vi "AxSyncLabVIEW.vi"() -> ()   [LabVIEW 2020]
panel:
  in  "Move position":i32
  in  "Refresh":bool
  in  "Tab Control":T1(tab)
  out "Analogue I/O":string
  out "Controller Type":string
  out "System Version":string
  out "Digital I/O":string
  out "Axis Parameters":string[][](table)
  in  "Axis":sgl
  out "HEX Representation of IO":string
  in  "WriteTable":bool
  in  "Entries":i32
  in  "Start":i32
  in  "Table Values":string[][](table)
  out "Table Size":dbl
  out "VR Values":string[][](table)
  in  "Start VR":ext
  in  "Entries VR":ext
  in  "Set VR":bool
  out "Directory Contents":string
  out "Status":string
  out "Axis Parameters 2":string[][](table)
  out "Watch Dog":bool
  in  "Run":bool
  out "CommPort":fxp<+,3,3>
  out "IsOpenLED":bool
  in  "Set Parameters":bool
  in  "Connection":string(combo)
  in  "Open/ Close":bool
  in  "stop":bool
  out "Error Out":errorcluster
  in  "Error In (no error)":errorcluster
  in  "Connection":refnum<k7>(container)
  # "WDOG OFF is illuminated\nas per coordinator"
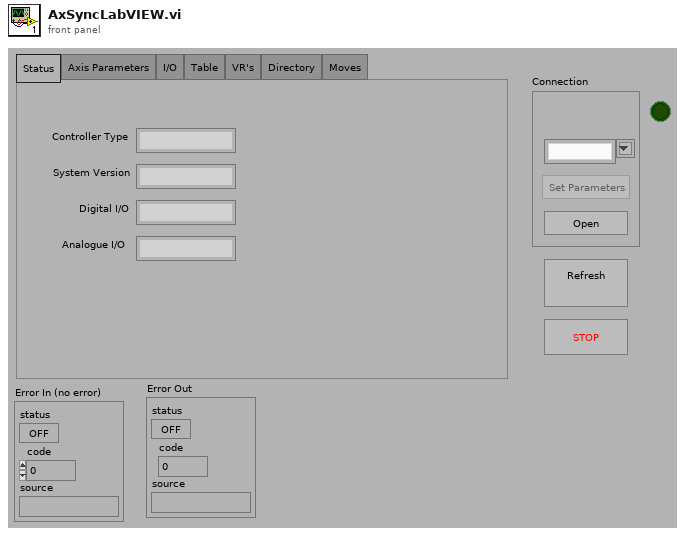
[diagram p1: front panel]
types:
  T1 = enum32{"Status", "Axis Parameters", "I/O", "Table", "VR's", "Directory", "Moves"}
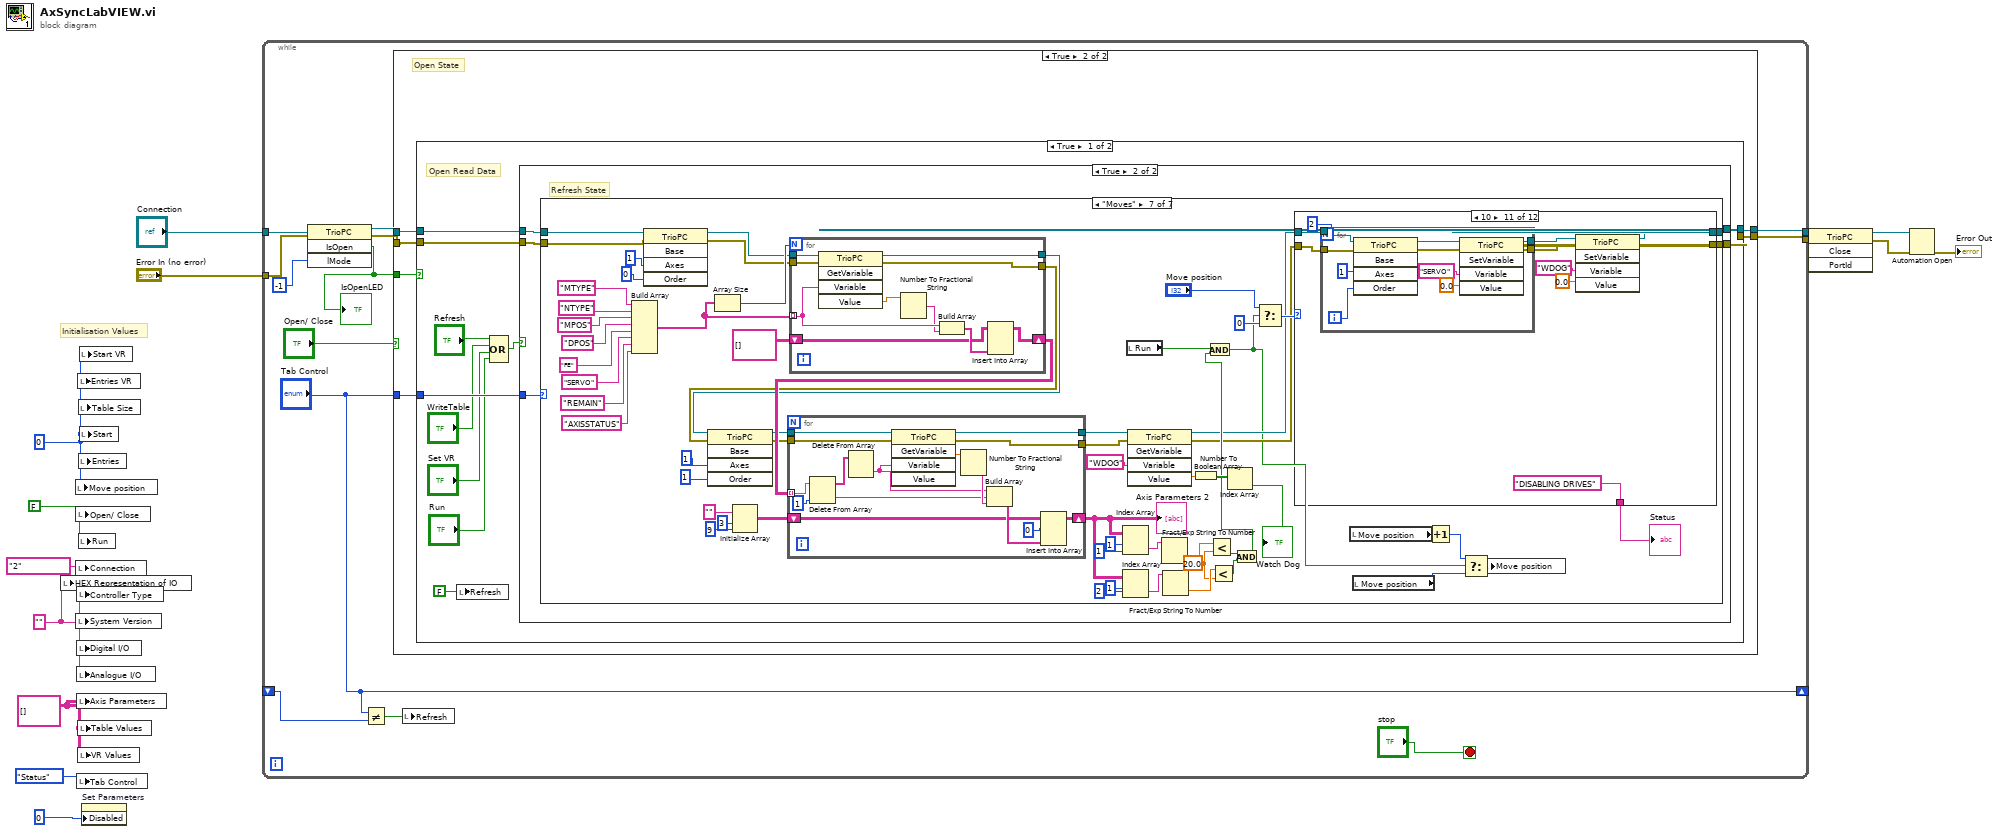
[diagram p0: block diagram]
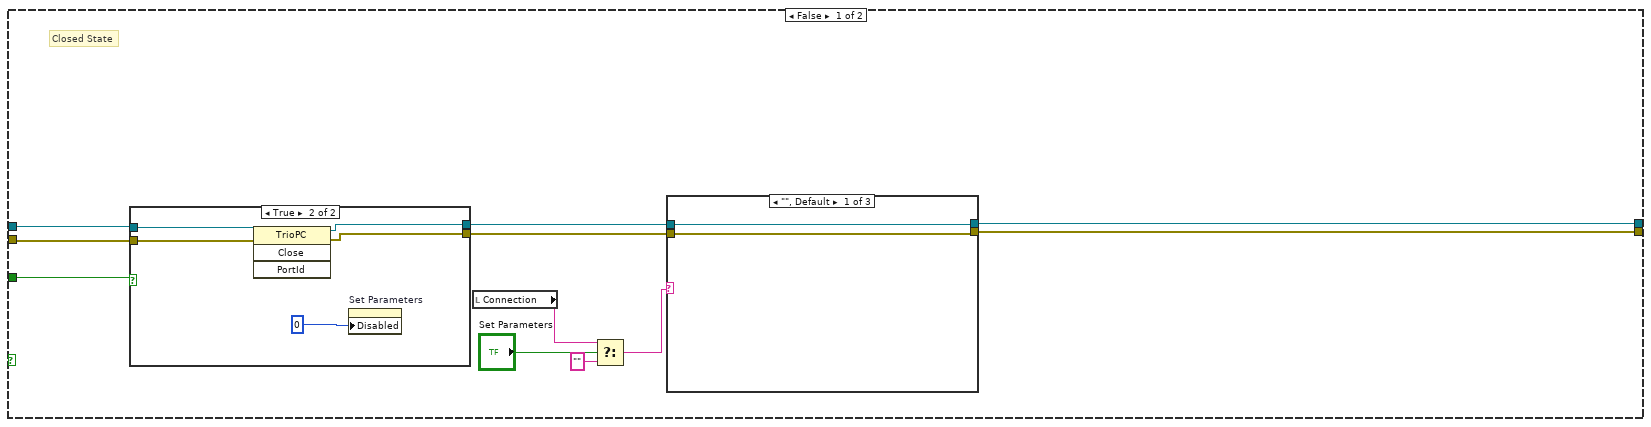
[diagram p2: hidden frame]
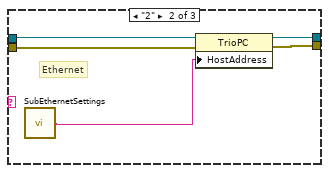
[diagram p3: hidden frame]
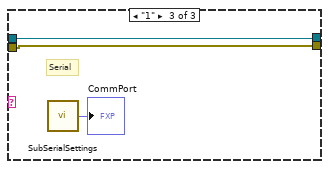
[diagram p4: hidden frame]
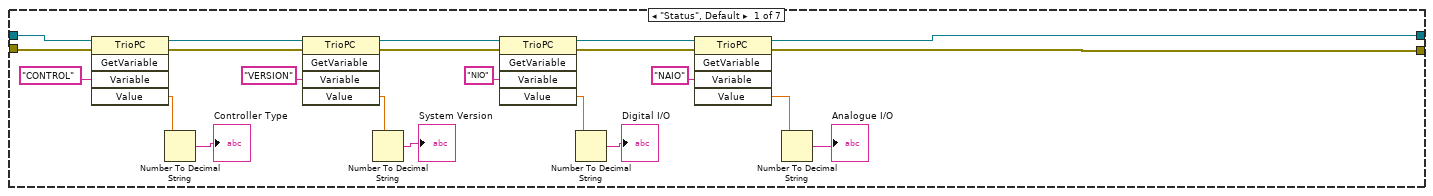
[diagram p7: hidden frame]
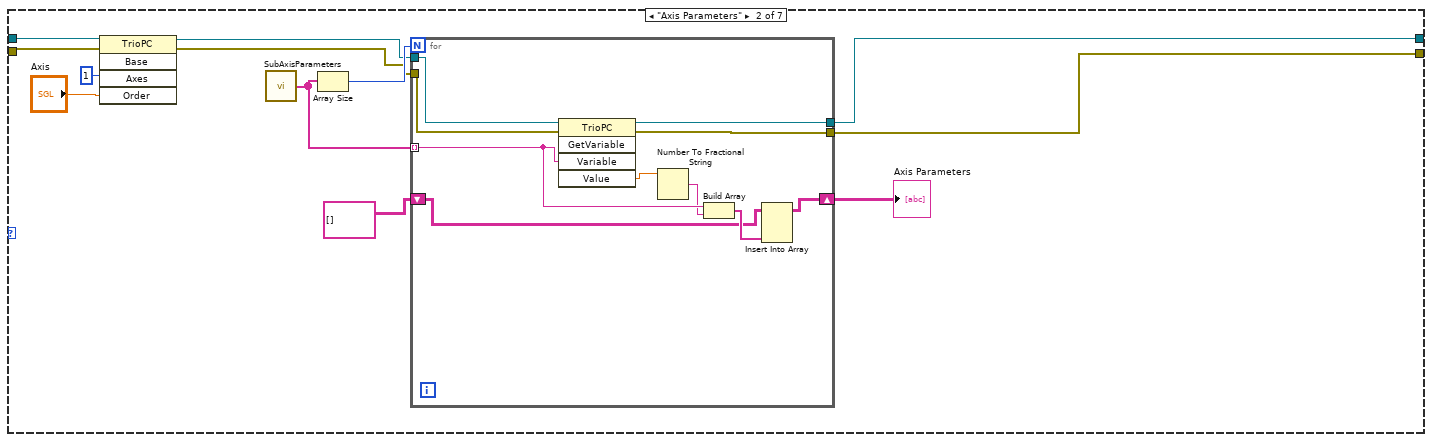
[diagram p8: hidden frame]
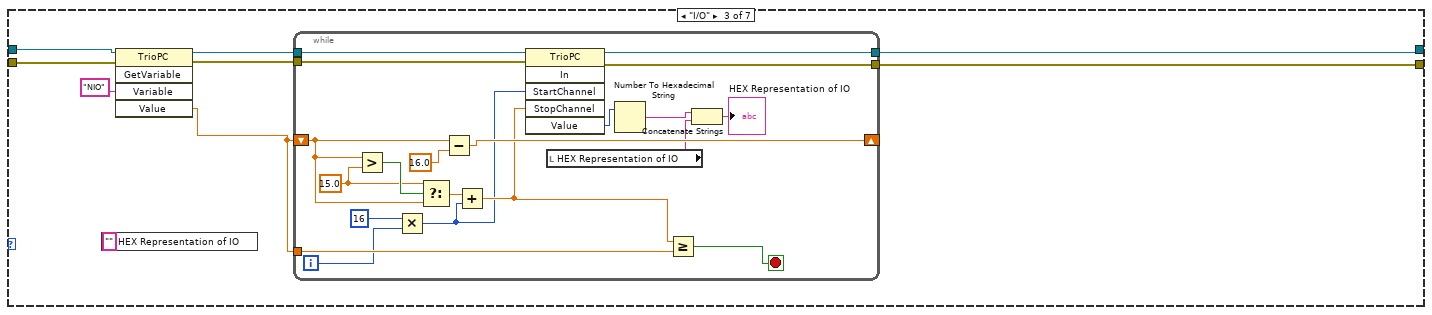
[diagram p9: hidden frame]
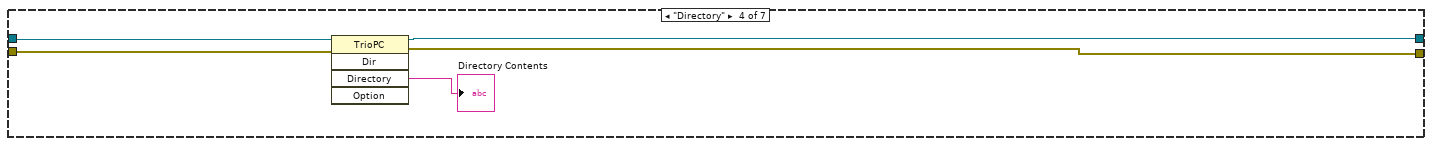
[diagram p10: hidden frame]
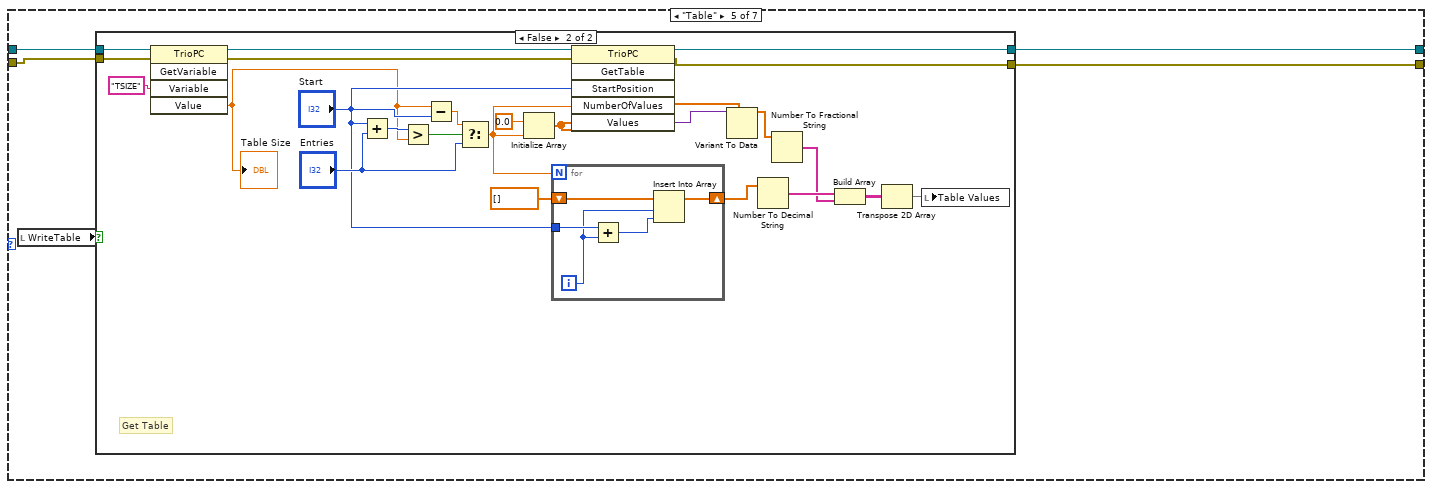
[diagram p11: hidden frame]
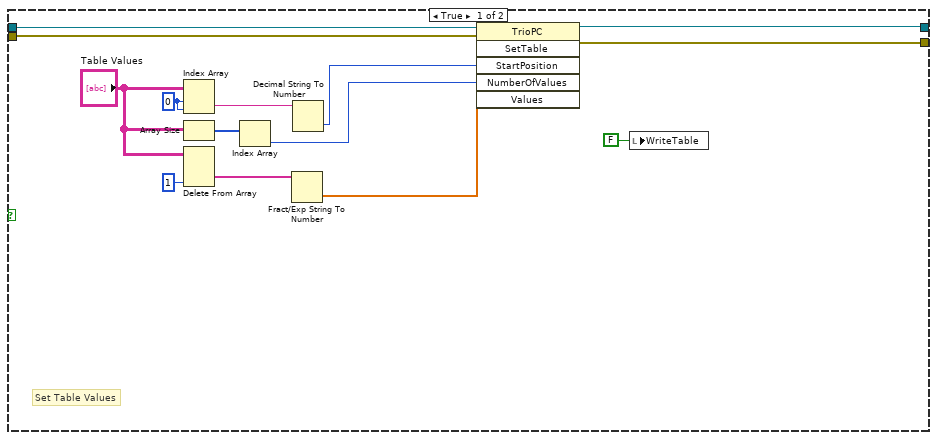
[diagram p12: hidden frame]
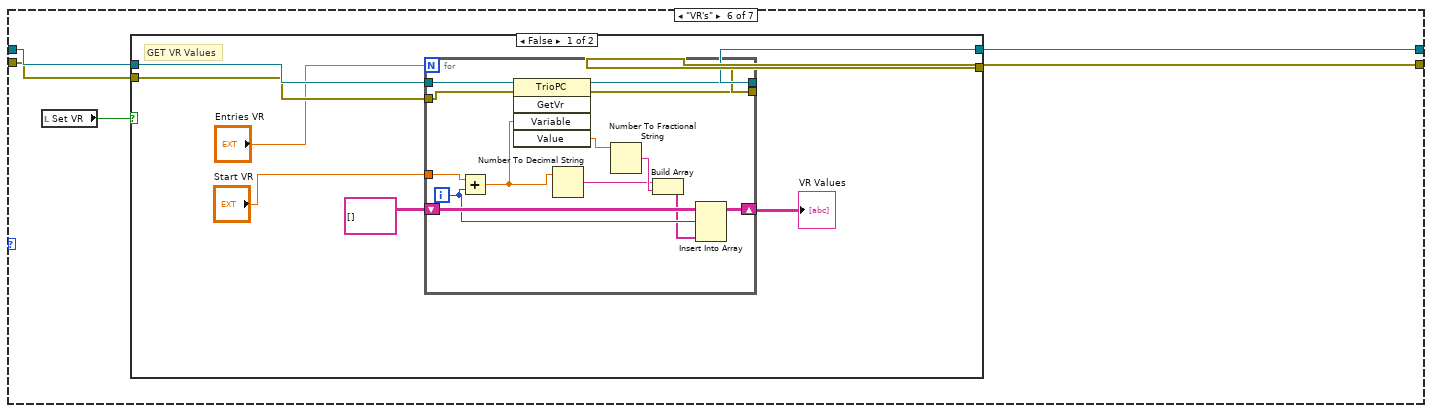
[diagram p13: hidden frame]
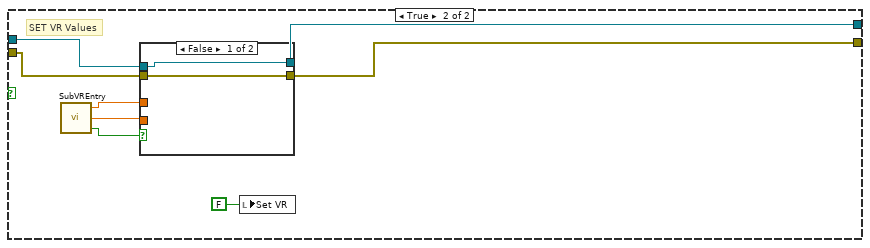
[diagram p14: hidden frame]
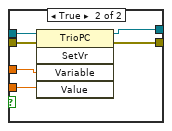
[diagram p15: hidden frame]
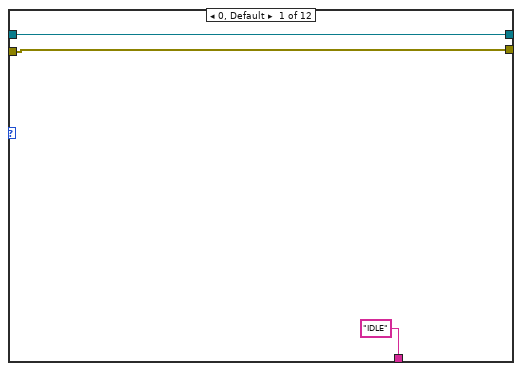
[diagram p16: hidden frame]
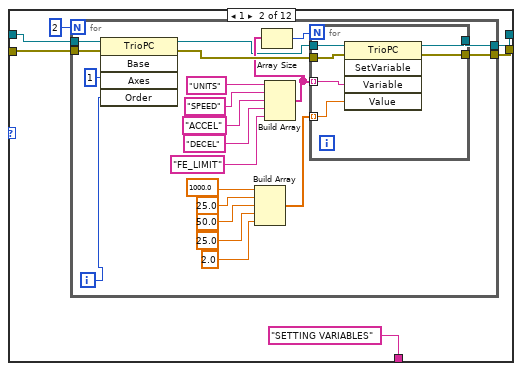
[diagram p17: hidden frame]
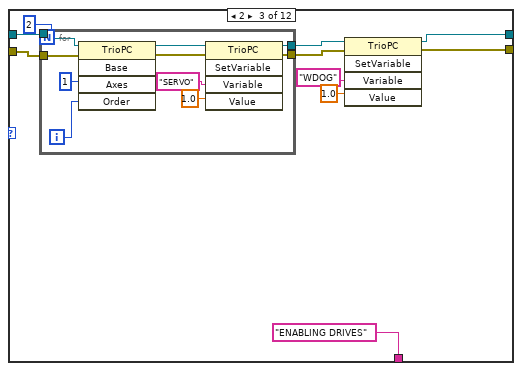
[diagram p18: hidden frame]
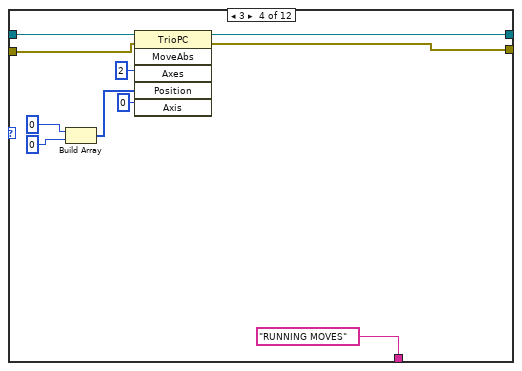
[diagram p19: hidden frame]
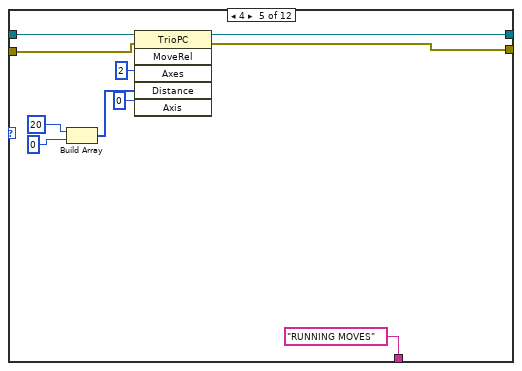
[diagram p20: hidden frame]
diagram:
  w4 = 0 ("Start")
  w8 = string[][] [] ("Axis Parameters")
  w1 = "" ("Controller Type")
  w3 = FALSE ("Open/ Close")
  # "Initialisation Values"
  n1 = local write "HEX Representation of IO"(w1) -> ()
  n2 = local write "Move position"(w4) -> ()
  n3 = local write "Open/ Close"(w3) -> ()
  n4 = local write "Connection"("2" ("Connection")) -> ()
  n5 = local write "System Version"(w1) -> ()
  n6 = local write "Controller Type"(w1) -> ()
  n7 = local write "Digital I/O"(w1) -> ()
  n8 = local write "Analogue I/O"(w1) -> ()
  n9 = local write "Axis Parameters"(w8) -> ()
  n10 = local write "Tab Control"(T1."Status" ("Tab Control")) -> ()
  n11 = local write "Entries VR"(w4) -> ()
  n12 = local write "Table Values"(w8) -> ()
  n13 = local write "VR Values"(w8) -> ()
  n14 = local write "Table Size"(w4) -> ()
  n15 = local write "Entries"(w4) -> ()
  n16 = local write "Run"(w3) -> ()
  n17 = local write "Start VR"(w4) -> ()
  n18 = local write "Start"(w4) -> ()
  n19 = property on="Set Parameters" class="Bool"("Disabled"=u8 0) -> ()  [unwired: 2 in, 2 out]
  n20 = while {
    tunnel: "Connection" -> [w21]
    tunnel: [w26] -> w6
    tunnel: "Error In (no error)" -> [w20]
    tunnel: [w25] -> w5
    shift-right: ["Tab Control"] -> _
    shift-left: _ -> [w17]
    stop <- "stop" stop-if-true
    n21 = invoke class="TrioPC" method="IsOpen"(reference=w21, error in=w20, "lMode"=-1) -> (reference out=w23:refnum<k7>, error out=w22:errorcluster, "IsOpen"=w19:bool)  [unwired: 1 in, 1 out]
    "IsOpenLED" <- w19
    n22 = Not Equal?(x="Tab Control", y=w17) -> (x != y?=w16:bool)
    n23 = case shown="True" "Open/ Close" {
      tunnel: w23 -> [w38 w59]
      tunnel: w22 -> [w37 w58]
      tunnel: [w30 w61] -> w26
      tunnel: [w28 w60] -> w25
      tunnel: w19 -> [w36 w57]
      tunnel: "Tab Control" -> [_ w56]
      frame False {
        # "Closed State"
        n24 = case shown="True" w36 {
          tunnel: w38 -> [w50 w55]
          tunnel: w37 -> [w49 w54]
          tunnel: [w50 w53] -> w32
          tunnel: [w49 w52] -> w31
          frame False {
          }
          frame True {
            n25 = invoke class="TrioPC" method="Close"(reference=w55, error in=w54) -> (reference out=w53:refnum<k7>, error out=w52:errorcluster)  [unwired: 2 in, 2 out]
            n26 = property on="Set Parameters" class="Bool"("Disabled"=u8 0) -> ()  [unwired: 2 in, 2 out]
          }
        }
        n27 = local read "Connection"() -> (w29:string)
        n28 = Select(t=w29, s="Set Parameters", f="") -> (s? t:f=w33:string)
        n29 = case shown="\"\", Default" w33 {
          tunnel: w32 -> [w40 w43 w48]
          tunnel: w31 -> [w39 w42 w47]
          tunnel: [w40 w45 w48] -> w30
          tunnel: [w39 w44 w47] -> w28
          frame "", Default {
          }
          frame "2" {
            # "Ethernet"
            n30 = call "SubEthernetSettings.vi"() -> ("Ethernet IP Address 2"=w41:string)
            n31 = property class="TrioPC"(reference=w43, error in=w42, "HostAddress"=w41) -> (reference out=w45:refnum<k7>, error out=w44:errorcluster)
          }
          frame "1" {
            # "Serial"
            n32 = call "SubSerialSettings.vi"() -> ("CommPort"=→"CommPort":fxp<+,3,3>)
          }
        }
      }
      frame True {
        # "Open State"
        n33 = case shown="True" w57 {
          tunnel: w59 -> [w72 w493]
          tunnel: w58 -> [w71 w492]
          tunnel: [w70 w491] -> w61
          tunnel: [w69 w490] -> w60
          tunnel: w56 -> [w68 _]
          frame True {
            # "Open Read Data"
            n34 = local write "Refresh"(FALSE ("Refresh")) -> ()
            n35 = Compound Arithmetic op=OR("Refresh", "WriteTable", "Set VR", "Run") -> (w66:bool)
            n36 = case shown="True" w66 {
              tunnel: w72 -> [w74 w79]
              tunnel: w71 -> [w73 w78]
              tunnel: [w74 w77] -> w70
              tunnel: [w73 w76] -> w69
              tunnel: w68 -> [_ w75]
              frame False {
                # "Idle State"
              }
              frame True {
                # "Refresh State"
                n37 = case shown="\"Moves\"" w75 {
                  tunnel: w79 -> [w101 w107 w131 w157 w160 w210 w298]
                  tunnel: w78 -> [w100 w106 w130 w156 w159 w209 w297]
                  tunnel: [w81 w109 w127 w155 w162 w207 w261] -> w77
                  tunnel: [w80 w110 w126 w154 w161 w206 w260] -> w76
                  frame "Status", Default {
                    n38 = invoke class="TrioPC" method="GetVariable"(reference=w101, error in=w100, "Variable"="CONTROL") -> (reference out=w95:refnum<k7>, error out=w94:errorcluster, "Value"=w89:dbl)  [unwired: 2 in, 2 out]
                    n39 = Number To Decimal String(number=w89) -> (decimal integer string=→"Controller Type":string)  [unwired: 1 in]
                    n40 = invoke class="TrioPC" method="GetVariable"(reference=w95, error in=w94, "Variable"="VERSION") -> (reference out=w93:refnum<k7>, error out=w92:errorcluster, "Value"=w87:dbl)  [unwired: 2 in, 2 out]
                    n41 = Number To Decimal String(number=w87) -> (decimal integer string=→"System Version":string)  [unwired: 1 in]
                    n42 = invoke class="TrioPC" method="GetVariable"(reference=w93, error in=w92, "Variable"="NIO") -> (reference out=w91:refnum<k7>, error out=w90:errorcluster, "Value"=w86:dbl)  [unwired: 2 in, 2 out]
                    n43 = Number To Decimal String(number=w86) -> (decimal integer string=→"Digital I/O":string)  [unwired: 1 in]
                    n44 = invoke class="TrioPC" method="GetVariable"(reference=w91, error in=w90, "Variable"="NAIO") -> (reference out=w81:refnum<k7>, error out=w80:errorcluster, "Value"=w85:dbl)  [unwired: 2 in, 2 out]
                    n45 = Number To Decimal String(number=w85) -> (decimal integer string=→"Analogue I/O":string)  [unwired: 1 in]
                  }
                  frame "Axis Parameters" {
                    n46 = invoke class="TrioPC" method="Base"(reference=w107, error in=w106, "Axes"=i16 1, "Order"="Axis") -> (reference out=w105:refnum<k7>, error out=w104:errorcluster)  [unwired: 1 in, 3 out]
                    n47 = call "SubAxisParameters.vi"() -> ("AxisParameters"=w113:string[])
                    n48 = Array Size(array=w113) -> (size(s)=w108:i32)
                    n49 = for {
                      N: w108 -> [_]
                      tunnel: w113 -> [w121] mode=indexing
                      tunnel: w105 -> [w123]
                      tunnel: w104 -> [w122]
                      shift-right: [w118] -> w112
                      shift-left: string[][] [] ("Axis Parameters") -> [w119]
                      tunnel: [w117] -> w109
                      tunnel: [w116] -> w110
                      n50 = invoke class="TrioPC" method="GetVariable"(reference=w123, error in=w122, "Variable"=w121) -> (reference out=w117:refnum<k7>, error out=w116:errorcluster, "Value"=w115:dbl)  [unwired: 2 in, 2 out]
                      n51 = Number To Fractional String(number=w115) -> (F-format string=w114:string)  [unwired: 3 in]
                      n52 = Build Array(w121, w114) -> (w120:string[])
                      n53 = Insert Into Array(array=w119, new element=w120) -> (w118:string[][])  [unwired: 2 in]
                    }
                    "Axis Parameters" <- w112
                  }
                  frame "I/O" {
                    n54 = local write "HEX Representation of IO"("" ("concatenated string")) -> ()
                    n55 = invoke class="TrioPC" method="GetVariable"(reference=w131, error in=w130, "Variable"="NIO") -> (reference out=w129:refnum<k7>, error out=w128:errorcluster, "Value"=w125:dbl)  [unwired: 2 in, 2 out]
                    n56 = while {
                      tunnel: w129 -> [w152]
                      tunnel: w128 -> [w151]
                      shift-right: [w148] -> _
                      shift-left: w125 -> [w142]
                      tunnel: [w147] -> w127
                      tunnel: [w146] -> w126
                      tunnel: w125 -> [w145]
                      i -> [w138]
                      stop <- w144 stop-if-true
                      w143 = 15.0 ("y")
                      n57 = Greater?(x=w142, y=w143) -> (0:w150:bool)
                      n58 = Multiply(x=16, y=w138) -> (x*y=w137:i32)
                      n59 = Select(t=w143, s=w150, f=w142) -> (s? t:f=w139:dbl)
                      n60 = Subtract(x=w142, y=16.0) -> (x-y=w148:dbl)
                      n61 = Add(x=w139, y=w137) -> (x+y=w140:dbl)
                      n62 = invoke class="TrioPC" method="In"(reference=w152, error in=w151, "StartChannel"=w137, "StopChannel"=w140) -> (reference out=w147:refnum<k7>, error out=w146:errorcluster, "Value"=w135:i32)  [unwired: 2 in, 3 out]
                      n63 = local read "HEX Representation of IO"() -> (w133:string)
                      n64 = Number To Hexadecimal String(2:w135) -> (0:w134:string)  [unwired: 1 in]
                      n65 = Greater Or Equal?(x=w140, y=w145) -> (x >= y?=w144:bool)
                      n66 = Concatenate Strings(w134, w133) -> (→"HEX Representation of IO":string)
                    }
                  }
                  frame "Directory" {
                    n67 = invoke class="TrioPC" method="Dir"(reference=w157, error in=w156) -> (reference out=w155:refnum<k7>, error out=w154:errorcluster, "Directory"=→"Directory Contents":string)  [unwired: 3 in, 2 out]
                  }
                  frame "Table" {
                    n68 = local read "WriteTable"() -> (w158:bool)
                    n69 = case shown="False" w158 {
                      tunnel: [w173 w199] -> w162
                      tunnel: [w172 w198] -> w161
                      tunnel: w160 -> [w174 w189]
                      tunnel: w159 -> [w175 w188]
                      frame True {
                        w176 = 0 ("index (row)")
                        # "Set Table Values"
                        n70 = Index Array(array="Table Values", index (row)=w176, index (col)=w176) -> (element=w171:string)
                        n71 = Array Size(array="Table Values") -> (size(s)=w169:i32[])
                        n72 = Delete From Array(array="Table Values", index (col)=1 ("disabled index (col)")) -> (deleted portion=w165:string[])  [unwired: 2 in, 1 out]
                        n73 = Index Array(array=w169) -> (element=w168:i32)  [unwired: 1 in]
                        n74 = Fract/Exp String To Number(string=w165) -> (number=w163:dbl[])  [unwired: 3 in, 1 out]
                        n75 = Decimal String To Number(string=w171) -> (number=w170:i32)  [unwired: 2 in, 1 out]
                        n76 = invoke class="TrioPC" method="SetTable"(reference=w174, error in=w175, "StartPosition"=w170, "NumberOfValues"=w168, "Values"=w163) -> (reference out=w173:refnum<k7>, error out=w172:errorcluster)  [unwired: 1 in, 4 out]
                        n77 = local write "WriteTable"(FALSE ("WriteTable")) -> ()
                      }
                      frame False {
                        # "Get Table"
                        n78 = invoke class="TrioPC" method="GetVariable"(reference=w189, error in=w188, "Variable"="TSIZE") -> (reference out=w187:refnum<k7>, error out=w186:errorcluster, "Value"=w177:dbl)  [unwired: 2 in, 2 out]
                        "Table Size" <- w177
                        n79 = Add(x="Start", y="Entries") -> (x+y=w184:i32)
                        n80 = Greater?(x=w184, y=w177) -> (0:w183:bool)
                        n81 = Subtract(x=w177, y="Start") -> (x-y=w179:dbl)
                        n82 = Select(t=w179, s=w183, f="Entries") -> (s? t:f=w181:dbl)
                        n83 = Initialize Array(0.0 ("disabled index (col)"), w181) -> (w195:dbl[])
                        n84 = for {
                          N: w181 -> [_]
                          shift-right: [w205] -> w193
                          shift-left: dbl[] [] -> [w204]
                          tunnel: "Start" -> [w203]
                          i -> [w201]
                          n85 = Add(x=w203, y=w201) -> (x+y=w202:i32)
                          n86 = Insert Into Array(array=w204, index=w201, new element=w202) -> (w205:dbl[])
                        }
                        n87 = invoke class="TrioPC" method="GetTable"(reference=w187, error in=w186, "StartPosition"="Start", "NumberOfValues"=w181, "Values"=w195) -> (reference out=w199:refnum<k7>, error out=w198:errorcluster, "Values"=w197:variant)  [unwired: 1 in, 3 out]
                        n88 = Variant To Data(type=w195, Variant=w197) -> (data=w191:dbl[])  [unwired: 1 in, 1 out]
                        n89 = Number To Decimal String(number=w193) -> (decimal integer string=w192:string[])  [unwired: 1 in]
                        n90 = Number To Fractional String(number=w191) -> (F-format string=w190:string[])  [unwired: 3 in]
                        n91 = Build Array(w192, w190) -> (w194:string[][])
                        n92 = Transpose 2D Array(2D array=w194) -> (transposed array=w178:string[][])
                        n93 = local write "Table Values"(w178) -> ()
                      }
                    }
                  }
                  frame "VR's" {
                    n94 = local read "Set VR"() -> (w208:bool)
                    n95 = case shown="False" w208 {
                      tunnel: w210 -> [w216 w239]
                      tunnel: [w218 w238] -> w207
                      tunnel: [w217 w237] -> w206
                      tunnel: w209 -> [w215 w236]
                      frame False {
                        # "GET VR Values"
                        n96 = for {
                          N: "Entries VR" -> [_]
                          tunnel: [w231] -> w218
                          tunnel: [w230] -> w217
                          tunnel: w216 -> [w229]
                          tunnel: w215 -> [w228]
                          tunnel: "Start VR" -> [w227]
                          shift-right: [w226] -> w213
                          shift-left: string[][] [] ("Axis Parameters") -> [w224]
                          i -> [w223]
                          n97 = Add(x=w227, y=w223) -> (x+y=w220:ext)
                          n98 = invoke class="TrioPC" method="GetVr"(reference=w229, error in=w228, "Variable"=w220) -> (reference out=w231:refnum<k7>, error out=w230:errorcluster, "Value"=w225:dbl)  [unwired: 2 in, 2 out]
                          n99 = Number To Decimal String(number=w220) -> (decimal integer string=w219:string)  [unwired: 1 in]
                          n100 = Number To Fractional String(number=w225) -> (F-format string=w222:string)  [unwired: 3 in]
                          n101 = Build Array(w219, w222) -> (w221:string[])
                          n102 = Insert Into Array(array=w224, index (row)=w223, new element=w221) -> (w226:string[][])  [unwired: 1 in]
                        }
                        "VR Values" <- w213
                      }
                      frame True {
                        # "SET VR Values"
                        n103 = call "SubVREntry.vi"() -> ("DataValid"=w233:bool, "Value 2"=w234:dbl, "VR 2"=w235:ext)
                        n104 = case shown="False" w233 {
                          tunnel: w239 -> [w241 w247]
                          tunnel: [w241 w246] -> w238
                          tunnel: [w240 w245] -> w237
                          tunnel: w236 -> [w240 w244]
                          tunnel: w235 -> [_ w243]
                          tunnel: w234 -> [_ w242]
                          frame False {
                          }
                          frame True {
                            n105 = invoke class="TrioPC" method="SetVr"(reference=w247, error in=w244, "Variable"=w243, "Value"=w242) -> (reference out=w246:refnum<k7>, error out=w245:errorcluster)  [unwired: 1 in, 3 out]
                          }
                        }
                        n106 = local write "Set VR"(FALSE ("Set VR")) -> ()
                      }
                    }
                  }
                  frame "Moves" {
                    w248 = 20.0 ("y")
                    n107 = Build Array("MTYPE", "NTYPE", "MPOS", "DPOS", "FE", "SERVO", "REMAIN", "AXISSTATUS") -> (w293:string[])
                    n108 = invoke class="TrioPC" method="Base"(reference=w298, error in=w297, "Axes"=i16 1, "Order"=i16 0 ("Axes")) -> (reference out=w296:refnum<k7>, error out=w294:errorcluster)  [unwired: 1 in, 3 out]
                    n109 = Array Size(array=w293) -> (size(s)=w308:i32)
                    n110 = Initialize Array("", 3 ("dimension size"), 9 ("dimension size")) -> (w286:string[][])
                    n111 = for {
                      N: w308 -> [_]
                      tunnel: w293 -> [w483] mode=indexing
                      tunnel: w296 -> [w484]
                      shift-right: [w480] -> w292
                      shift-left: string[][] [] ("Axis Parameters") -> [w481]
                      tunnel: [w479] -> w288
                      tunnel: [w475] -> w287
                      tunnel: w294 -> [w476]
                      n112 = invoke class="TrioPC" method="GetVariable"(reference=w484, error in=w476, "Variable"=w483) -> (reference out=w479:refnum<k7>, error out=w475:errorcluster, "Value"=w478:dbl)  [unwired: 2 in, 2 out]
                      n113 = Number To Fractional String(number=w478) -> (F-format string=w477:string)  [unwired: 3 in]
                      n114 = Build Array(w483, w477) -> (w482:string[])
                      n115 = Insert Into Array(array=w481, new element=w482) -> (w480:string[][])  [unwired: 2 in]
                    }
                    n116 = invoke class="TrioPC" method="Base"(reference=w288, error in=w287, "Axes"=i16 1, "Order"=i16 1 ("Axes")) -> (reference out=w290:refnum<k7>, error out=w289:errorcluster)  [unwired: 1 in, 3 out]
                    n117 = for {
                      tunnel: w292 -> [w468] mode=indexing
                      tunnel: w290 -> [w474]
                      tunnel: [w473] -> w280
                      tunnel: [w472] -> w279
                      tunnel: w289 -> [w470]
                      shift-right: [w460] -> w274
                      shift-left: w286 -> [w461]
                      n118 = Delete From Array(array=w468, index=1) -> (deleted portion=w466:string, array with subset deleted=w465:string[])  [unwired: 1 in]
                      n119 = Delete From Array(array=w465) -> (deleted portion=w464:string)  [unwired: 2 in, 1 out]
                      n120 = invoke class="TrioPC" method="GetVariable"(reference=w474, error in=w470, "Variable"=w464) -> (reference out=w473:refnum<k7>, error out=w472:errorcluster, "Value"=w471:dbl)  [unwired: 2 in, 2 out]
                      n121 = Number To Fractional String(number=w471) -> (F-format string=w469:string)  [unwired: 3 in]
                      n122 = Build Array(w464, w466, w469) -> (w463:string[])
                      n123 = Insert Into Array(array=w461, index (row)=0, new element=w463) -> (w460:string[][])  [unwired: 1 in]
                    }
                    "Axis Parameters 2" <- w274
                    n124 = Index Array(array=w274, index (row)=1, index (col)=1 ("disabled index (col)")) -> (element=w269:string)
                    n125 = Index Array(array=w274, index (row)=1, index (col)=2 ("disabled index (col)")) -> (element=w268:string)
                    n126 = local read "Run"() -> (w267:bool)
                    n127 = invoke class="TrioPC" method="GetVariable"(reference=w280, error in=w279, "Variable"="WDOG") -> (reference out=w262:refnum<k7>, error out=w259:errorcluster, "Value"=w277:dbl)  [unwired: 2 in, 2 out]
                    n128 = Fract/Exp String To Number(string=w269) -> (number=w251:dbl)  [unwired: 3 in, 1 out]
                    n129 = Fract/Exp String To Number(string=w268) -> (number=w249:dbl)  [unwired: 3 in, 1 out]
                    n130 = Number To Boolean Array(number=w277) -> (Boolean array=w276:bool[])
                    n131 = Less?(x=w251, y=w248) -> (x < y?=w252:bool)
                    n132 = Less?(x=w249, y=w248) -> (x < y?=w250:bool)
                    n133 = Index Array(array=w276) -> (element=→"Watch Dog":bool)  [unwired: 1 in]
                    n134 = And(x=w252, y=w250) -> (x .and. y?=w266:bool)
                    n135 = And(x=w267, y=w266) -> (x .and. y?=w254:bool)
                    n136 = Select(t="Move position", s=w254, f=0) -> (s? t:f=w265:i32)
                    n137 = case shown="10" w265 {
                      tunnel: w262 -> [w311 w315 w350 w374 w384 w394 w404 w414 w424 w434 w440 w457]
                      tunnel: [w311 w317 w352 w373 w383 w393 w403 w413 w423 w433 w442 w457] -> w261
                      tunnel: w259 -> [w310 w314 w349 w371 w381 w391 w401 w411 w421 w431 w439 w456]
                      tunnel: [w310 w316 w351 w372 w382 w392 w402 w412 w422 w432 w441 w456] -> w260
                      tunnel: ["IDLE" ("Status") "SETTING VARIABLES" ("Status") "ENABLING DRIVES" ("Status") "RUNNING MOVES" ("Status") "RUNNING MOVES" ("Status") "RUNNING MOVES" ("Status") "RUNNING MOVES" ("Status") "RUNNING MOVES" ("Status") "RUNNING MOVES" ("Status") "RUNNING MOVES" ("Status") "DISABLING DRIVES" ("Status") "IDLE" ("Status")] -> w253
                      frame 0, Default {
                      }
                      frame 1 {
                        n138 = for {
                          N: 2 -> [_]
                          tunnel: [w338] -> w317
                          tunnel: [w337] -> w316
                          tunnel: w315 -> [w325]
                          tunnel: w314 -> [w324]
                          i -> [w318]
                          n139 = invoke class="TrioPC" method="Base"(reference=w325, error in=w324, "Axes"=i16 1, "Order"=w318) -> (reference out=w321:refnum<k7>, error out=w323:errorcluster)  [unwired: 1 in, 3 out]
                          n140 = Build Array(1000.0 ("Value"), 25.0 ("Value"), 50.0 ("Value"), 25.0 ("Value"), 2.0 ("Value")) -> (w326:dbl[])
                          n141 = Build Array("UNITS" ("Variable"), "SPEED" ("Variable"), "ACCEL" ("Variable"), "DECEL" ("Variable"), "FE_LIMIT" ("Variable")) -> (w322:string[])
                          n142 = Array Size(array=w322) -> (size(s)=w320:i32)
                          n143 = for {
                            N: w320 -> [_]
                            tunnel: [w344] -> w338
                            tunnel: [w343] -> w337
                            tunnel: w321 -> [w342]
                            tunnel: w323 -> [w341]
                            tunnel: w322 -> [w340] mode=indexing
                            tunnel: w326 -> [w339] mode=indexing
                            n144 = invoke class="TrioPC" method="SetVariable"(reference=w342, error in=w341, "Variable"=w340, "Value"=w339) -> (reference out=w344:refnum<k7>, error out=w343:errorcluster)  [unwired: 1 in, 3 out]
                          }
                        }
                      }
                      frame 2 {
                        n145 = for {
                          N: 2 -> [_]
                          tunnel: [w364] -> w354
                          tunnel: [w363] -> w353
                          tunnel: w350 -> [w358]
                          tunnel: w349 -> [w357]
                          i -> [w355]
                          n146 = invoke class="TrioPC" method="Base"(reference=w358, error in=w357, "Axes"=i16 1, "Order"=w355) -> (reference out=w360:refnum<k7>, error out=w359:errorcluster)  [unwired: 1 in, 3 out]
                          n147 = invoke class="TrioPC" method="SetVariable"(reference=w360, error in=w359, "Variable"="SERVO", "Value"=1.0) -> (reference out=w364:refnum<k7>, error out=w363:errorcluster)  [unwired: 1 in, 3 out]
                        }
                        n148 = invoke class="TrioPC" method="SetVariable"(reference=w354, error in=w353, "Variable"="WDOG", "Value"=1.0) -> (reference out=w352:refnum<k7>, error out=w351:errorcluster)  [unwired: 1 in, 3 out]
                      }
                      frame 3 {
                        n149 = Build Array(0, 0) -> (w367:i32[])
                        n150 = invoke class="TrioPC" method="MoveAbs"(reference=w374, error in=w371, "Axes"=i16 2, "Position"=w367, "Axis"=i16 0 ("Axes")) -> (reference out=w373:refnum<k7>, error out=w372:errorcluster)  [unwired: 1 in, 4 out]
                      }
                      frame 4 {
                        n151 = Build Array(20, 0) -> (w377:i32[])
                        n152 = invoke class="TrioPC" method="MoveRel"(reference=w384, error in=w381, "Axes"=i16 2, "Distance"=w377, "Axis"=i16 0 ("Axes")) -> (reference out=w383:refnum<k7>, error out=w382:errorcluster)  [unwired: 1 in, 4 out]
                      }
                      frame 5 {
                        n153 = Build Array(-20, -50) -> (w387:i32[])
                        n154 = invoke class="TrioPC" method="MoveRel"(reference=w394, error in=w391, "Axes"=i16 2, "Distance"=w387, "Axis"=i16 0 ("Axes")) -> (reference out=w393:refnum<k7>, error out=w392:errorcluster)  [unwired: 1 in, 4 out]
                      }
                      frame 6 {
                        n155 = Build Array(-20, 50) -> (w397:i32[])
                        n156 = invoke class="TrioPC" method="MoveRel"(reference=w404, error in=w401, "Axes"=i16 2, "Distance"=w397, "Axis"=i16 0 ("Axes")) -> (reference out=w403:refnum<k7>, error out=w402:errorcluster)  [unwired: 1 in, 4 out]
                      }
                      frame 7 {
                        n157 = Build Array(20, 50) -> (w407:i32[])
                        n158 = invoke class="TrioPC" method="MoveRel"(reference=w414, error in=w411, "Axes"=i16 2, "Distance"=w407, "Axis"=i16 0 ("Axes")) -> (reference out=w413:refnum<k7>, error out=w412:errorcluster)  [unwired: 1 in, 4 out]
                      }
                      frame 8 {
                        n159 = Build Array(20, -50) -> (w417:i32[])
                        n160 = invoke class="TrioPC" method="MoveRel"(reference=w424, error in=w421, "Axes"=i16 2, "Distance"=w417, "Axis"=i16 0 ("Axes")) -> (reference out=w423:refnum<k7>, error out=w422:errorcluster)  [unwired: 1 in, 4 out]
                      }
                      frame 9 {
                        n161 = Build Array(0, 0) -> (w428:i32[])
                        n162 = invoke class="TrioPC" method="MoveAbs"(reference=w434, error in=w431, "Axes"=i16 2, "Position"=w428, "Axis"=i16 0 ("Axes")) -> (reference out=w433:refnum<k7>, error out=w432:errorcluster)  [unwired: 1 in, 4 out]
                      }
                      frame 10 {
                        n163 = for {
                          N: 2 -> [_]
                          tunnel: [w454] -> w444
                          tunnel: [w453] -> w443
                          tunnel: w440 -> [w448]
                          tunnel: w439 -> [w447]
                          i -> [w445]
                          n164 = invoke class="TrioPC" method="Base"(reference=w448, error in=w447, "Axes"=i16 1, "Order"=w445) -> (reference out=w450:refnum<k7>, error out=w449:errorcluster)  [unwired: 1 in, 3 out]
                          n165 = invoke class="TrioPC" method="SetVariable"(reference=w450, error in=w449, "Variable"="SERVO", "Value"=0.0) -> (reference out=w454:refnum<k7>, error out=w453:errorcluster)  [unwired: 1 in, 3 out]
                        }
                        n166 = invoke class="TrioPC" method="SetVariable"(reference=w444, error in=w443, "Variable"="WDOG", "Value"=0.0) -> (reference out=w442:refnum<k7>, error out=w441:errorcluster)  [unwired: 1 in, 3 out]
                      }
                      frame 11 {
                        n167 = local write "Move position"(0 ("Move position")) -> ()
                        n168 = local write "Run"(FALSE ("Run")) -> ()
                      }
                    }
                    "Status" <- w253
                    n169 = local read "Move position"() -> (w258:i32)
                    n170 = local read "Move position"() -> (w255:i32)
                    n171 = Increment(x=w258) -> (x+1=w256:i32)
                    n172 = Select(t=w256, s=w254, f=w255) -> (s? t:f=w257:i32)
                    n173 = local write "Move position"(w257) -> ()
                  }
                }
              }
            }
          }
          frame False {
            # "Opening State"
            n174 = Decimal String To Number(string="Connection") -> (number=w494:i32)  [unwired: 2 in, 1 out]
            n175 = case shown="2" w494 {
              tunnel: [i16 0 ("PortId") w497 i16 3240 ("PortId")] -> w495
              frame 0, Default {
              }
              frame 1 {
                n176 = local read "CommPort"() -> (w497:fxp<+,3,3>)
              }
              frame 2 {
              }
            }
            n177 = invoke class="TrioPC" method="Open"(reference=w493, error in=w492, "PortType"=w494, "PortId"=w495) -> (reference out=w491:refnum<k7>, error out=w490:errorcluster, "Open"=w485:bool)  [unwired: 1 in, 2 out]
            n178 = Select(t=u8 2, s=w485, f=u8 0 ("Disabled")) -> (s? t:f=w486:u8)
            n179 = local write "Open/ Close"(w485) -> ()
            n180 = property on="Set Parameters" class="Bool"("Disabled"=w486) -> ()  [unwired: 2 in, 2 out]
          }
        }
      }
    }
    n181 = local write "Refresh"(w16) -> ()
  }
  n182 = invoke class="TrioPC" method="Close"(reference=w6, error in=w5) -> (reference out=w13:refnum<k7>, error out=w12:errorcluster)  [unwired: 2 in, 2 out]
  n183 = Automation Open(error in (no error)=w12, Automation Refnum=w13) -> (error out=→"Error Out":errorcluster)  [unwired: 2 in, 1 out]
